vi "Read Process Variables.vi"(7 "Unit Address (1)":u8=1, 8 "error in (no error)":errorcluster, 11 "VISA resource name":refnum<visa-resource-name>) -> (0 "error out":errorcluster, 1 "Measured Value":i16, 2 "Process Value":i16, 3 "VISA resource name out":refnum<visa-resource-name>)   [LabVIEW 2014, in "Eurotherm 35xx Series.lvlib"]
doc: "This VI returns Process Value and associated variable."
uses:
  <instrlib>/Eurotherm 35xx Series/Eurotherm 35xx Series.lvlib
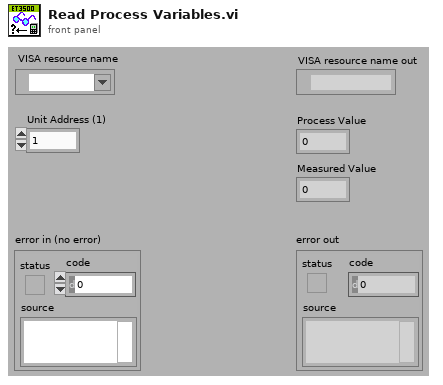
[diagram p1: front panel]
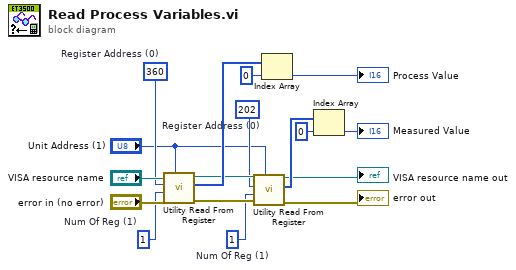
[diagram p0: block diagram]
diagram:
  w6 = u16 1  # Num Of Reg (1)
  w9 = u16 202  # Register Address (0)
  w14 = u16 360  # Register Address (0)
  w15 = u16 1  # Num Of Reg (1)
  n1 = call <instrlib>:"Utility Read From Register.vi"("Unit Address (1)"="Unit Address (1)", "error in (no error)"="error in (no error)", "Num Of Reg (1)"=w15, "Register Address (0)"=w14, "VISA resource name"="VISA resource name") -> ("error out"=w11:errorcluster, "Data"=w13:i16[], "VISA resource name out"=w10:refnum<visa-resource-name>)  [unwired: 4 in]
  n2 = call <instrlib>:"Utility Read From Register.vi"("Unit Address (1)"="Unit Address (1)", "error in (no error)"=w11, "Num Of Reg (1)"=w6, "Register Address (0)"=w9, "VISA resource name"=w10) -> ("error out"=→"error out":errorcluster, "Data"=w7:i16[], "VISA resource name out"=→"VISA resource name out":refnum<visa-resource-name>)  [unwired: 4 in]
  n3 = Index Array(array=w13, index=0) -> (element=→"Process Value":i16)
  n4 = Index Array(array=w7, index=0) -> (element=→"Measured Value":i16)
